vi "add keypair mem.vi"(8 "error in":errorcluster, 9 "key":string, 10 "cert":string, 11 "lvlibretls server listener in":refnum<class "lvlibretls server listener.lvclass">) -> (0 "error out":errorcluster, 3 "lvlibretls server listener out":refnum<class "lvlibretls server listener.lvclass">)   [LabVIEW 2016, in "lvlibretls server listener.lvclass"]
uses:
  lvlibretls server listener.lvclass
  C:/Users/IEUser/Desktop/tlssimple/lvlibtls/context parent/lvlibretls configurable context.lvclass
  context parent/lvlibretls configurable context.lvclass/lvlibretls configurable context.ctl
  context parent/lvlibretls configurable context.lvclass
  lv tls dll.lvlib
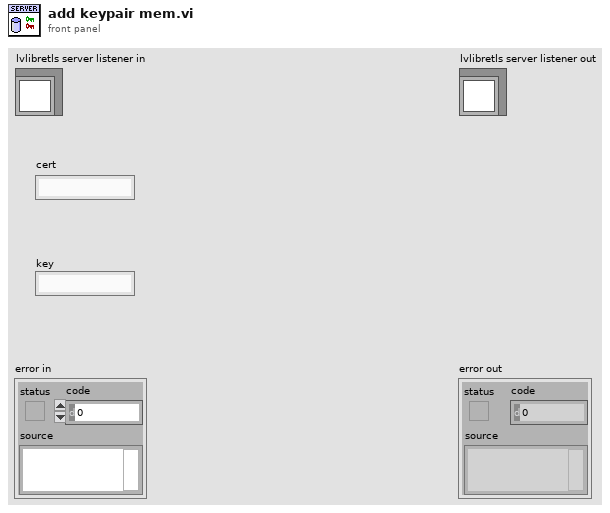
[diagram p1: front panel]
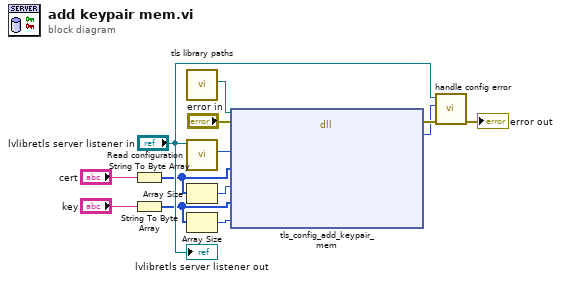
[diagram p0: block diagram]
diagram:
  n1 = String To Byte Array(string="cert") -> (unsigned byte array=w4:u8[])
  n2 = String To Byte Array(string="key") -> (unsigned byte array=w5:u8[])
  n3 = call "tls library paths.vi"() -> ("libtls"=w12:path)  [unwired: 8 in, 3 out]
  n4 = call "Read configuration.vi"("lvlibretls configurable context in"="lvlibretls server listener in") -> ("configuration"=w11:u64)  [unwired: 10 in]
  n5 = Array Size(array=w4) -> (size(s)=w3:i32)
  n6 = Array Size(array=w5) -> (size(s)=w2:i32)
  n7 = dll-call lib="C:/Users/IEUser/Desktop/tlssimple/libtls-15.dll" fn="tls_config_add_keypair_mem"(path in=w12, error in="error in", "config"=w11, "cert"=w4, "cert len"=w3, "key"=w5, "key len"=w2) -> (error out=w10:errorcluster, "return"=w1:i32)  [unwired: 6 in, 1 out]
  n8 = call "handle config error.vi"("error in"=w10, "return"=w1, "lvlibretls configurable context in"="lvlibretls server listener in") -> ("error out"=→"error out":errorcluster)  [unwired: 8 in]
  "lvlibretls server listener out" <- "lvlibretls server listener in"
